vi "Write Frame (DBDE) (SubVI).vi"(5 "Data":T1, 8 "Record":bool, 11 "FILE REF IN":refnum<file>) -> (3 "FILE REF OUT":refnum<file>)   [LabVIEW 2015]
uses:
  Controls (HOST)/Data to Disk Bundle.ctl
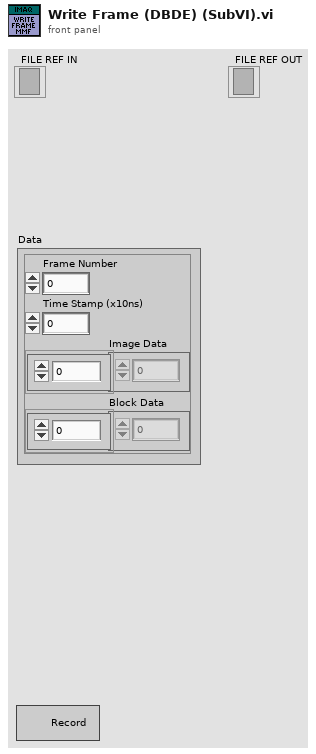
[diagram p1: front panel]
types:
  T1 = typedef "Data to Disk Bundle.ctl" = cluster{"Frame Number":u64, "Time Stamp (x10ns)":u64, "Image Data":u64[], "Block Data":u64[]}
  T2 = enum16{"big-endian, network order", "native, host order", "little-endian"}
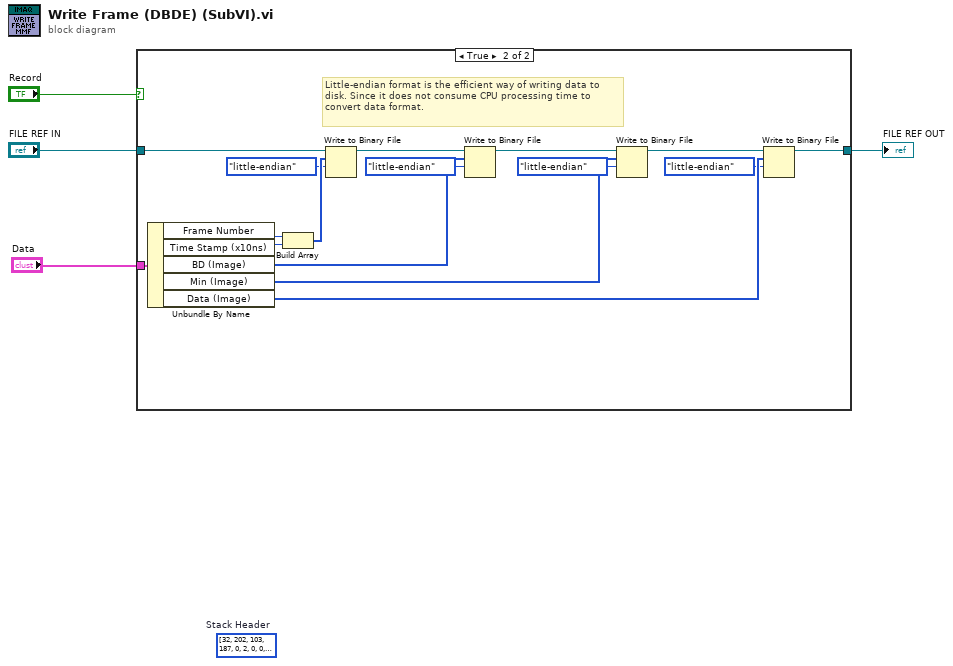
[diagram p0: block diagram]
diagram:
  (unwired) u8[] [32, 202, 103, 187, 0, 2, 0, 0, 90, 243, 155, 0, 180, 0, 0, 0, 0, 0, 0, 0, 0, 0, 0, 0, 0, 0, 0, 0, 0, 0, 0, 0, 0, 0, 0, 0, 0, 0, 0, 0, 0, 0, 0, 0, 0, 0, 0, 0, 0, 0, 0, 0, 0, 0, 0, 0, 0, 0, 0, 0, 0, 0, 0, 0, 0, 0, 0, 0, 0, 0, 0, 0, 0, 0, 0, 0, 0, 0, 0, 0, 0, 0, 0, 0, 0, 0, 0, 0, 0, 0, 0, 0, 0, 0, 0, 0, 0, 0, 0, 0, 0, 0, 0, 0, 0, 0, 0, 0, 0, 0, 0, 0, 0, 0, 0, 0, 0, 0, 0, 0, 0, 0, 0, 0, 0, 0, 0, 0, 0, 0, 0, 0, 0, 0, 0, 0, 0, 0, 0, 0, 0, 0, 0, 0, 0, 0, 0, 0, 0, 0, 0, 0, 0, 0, 0, 0, 0, 0, 0, 0, 0, 0, 0, 0, 0, 0, 0, 0, 0, 0, 0, 0, 0, 0, 0, 0, 0, 0, 0, 0, 0, 0, 0, 0, 0, 0, 0, 0, 0, 0, 0, 0, 0, 0, 0, 0, 0, 0, 0, 0, 0, 0, 0, 0, 0, 0, 0, 0, 0, 0, 0, 0, 0, 0, 0, 0, 0, 0, 0, 0, 0, 0, 0, 0, 0, 0, 0, 0, 0, 0, 0, 0, 0, 0, 0, 0, 0, 0, 0, 0, 0, 0, 0, 0, 0, 0, 0, 0, 0, 0, 0, 0, 0, 0, 0, 0, 0, 0, 0, 0, 0, 0, 0, 0, 0, 0, 0, 0, 0, 0, 0, 0, 0, 0, 0, 0, 0, 0, 0, 0, 0, 0, 0, 0, 0, 0, 0, 0, 0, 0, 0, 0, 0, 0, 0, 0, 0, 0, 0, 0, 0, 0, 0, 0, 0, 0, 0, 0, 0, 0, 0, 0, 0, 0, 0, 0, 0, 0, 0, 0, 0, 0, 0, 0, 0, 0, 0, 0, 0, 0, 0, 0, 0, 0, 0, 0, 0, 0, 0, 0, 0, 0, 0, 0, 0, 0, 0, 0, 0, 0, 0, 0, 0, 0, 0, 0, 0, 0, 0, 0, 0, 0, 0, 0, 0, 0, 0, 0, 0, 0, 0, 0, 0, 0, 0, 0, 0, 0, 0, 0, 0, 0, 0, 0, 0, 0, 0, 0, 0, 0, 0, 0, 0, 0, 0, 0, 0, 0, 0, 0, 0, 0, 0, 0, 0, 0, 0, 0, 0, 0, 0, 0, 0, 0, 0, 0, 0, 0, 0, 0, 0, 0, 0, 0, 0, 0, 0, 0, 0, 0, 0, 0, 0, 0, 0, 0, 0, 0, 0, 0, 0, 0, 0, 0, 0, 0, 0, 0, 0, 0, 0, 0, 0, 0, 0, 0, 0, 0, 0, 0, 0, 0, 0, 0, 0, 0, 0, 0, 0, 0, 0, 0, 0, 0, 0, 0, 0, 0, 0, 0, 0, 0, 0, 0, 0, 0, 0, 0, 0, 0, 0, 0, 0, 0, 0, 0, 0, 0, 0, 0, 0, 0, 0, 0, 0, 0, 0, 0, 0, 0, 0, 0]  # Stack Header
  n1 = case shown="True" "Record" {
    tunnel: [w5 w16] -> w4
    tunnel: "FILE REF IN" -> [w5 w21]
    tunnel: "Data" -> [_ w19]
    frame False {
    }
    frame True {
      # "Little-endian format is the efficient way of writing data to disk. Since it does not consume CPU processing time to convert data format."
      n2 = Unbundle By Name(w19) -> ("Frame Number"=w15:u64, "Time Stamp (x10ns)"=w14:u64, "BD (Image)"=w12:u8[], "Min (Image)"=w11:u8[], "Data (Image)"=w10:u64[])
      n3 = Build Array(w15, w14) -> (w13:u64[])
      n4 = Write to Binary File(file (use dialog)=w21, data=w13, 9:T2."little-endian" ("byte order (0:big-endian, network order)")) -> (refnum out=w20:refnum<file>)  [unwired: 3 in, 2 out]
      n5 = Write to Binary File(file (use dialog)=w20, data=w12, 9:T2."little-endian" ("byte order (0:big-endian, network order)")) -> (refnum out=w18:refnum<file>)  [unwired: 3 in, 2 out]
      n6 = Write to Binary File(file (use dialog)=w18, data=w11, 9:T2."little-endian" ("byte order (0:big-endian, network order)")) -> (refnum out=w17:refnum<file>)  [unwired: 3 in, 2 out]
      n7 = Write to Binary File(file (use dialog)=w17, data=w10, 9:T2."little-endian" ("byte order (0:big-endian, network order)")) -> (refnum out=w16:refnum<file>)  [unwired: 3 in, 2 out]
    }
  }
  "FILE REF OUT" <- w4
